vi "SetNeoPixelColourRing.vi"(8 "error in (no error)":errorcluster, 10 "NeoPixel Ring in":T1, 11 "AdaFruit-Seesaw in":refnum<class "AdaFruit-Seesaw.lvclass">) -> (0 "error out":errorcluster, 3 "AdaFruit-Seesaw out":refnum<class "AdaFruit-Seesaw.lvclass">)   [LabVIEW 2020, in "CTI-Scratchpad.lvlib"]
uses:
  CTI-Scratchpad.lvlib
  CTI-Peripheral/AdaFruit-Seesaw/AdaFruit-Seesaw.lvclass
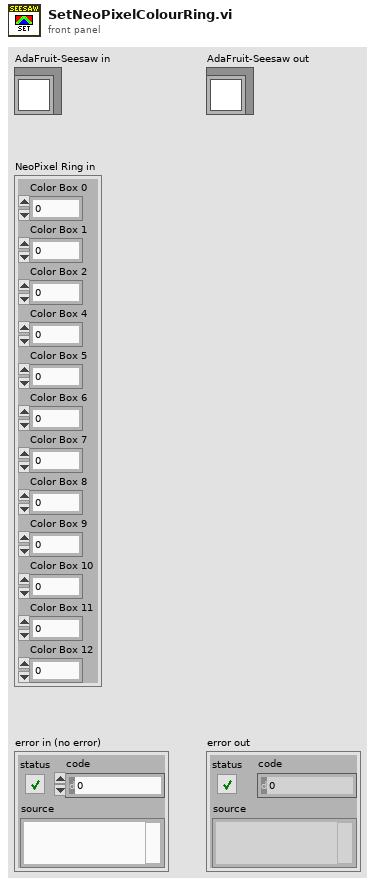
[diagram p1: front panel]
types:
  T1 = cluster{"Color Box 0":u32, "Color Box 1":u32, "Color Box 2":u32, "Color Box 4":u32, "Color Box 5":u32, "Color Box 6":u32, "Color Box 7":u32, "Color Box 8":u32, "Color Box 9":u32, "Color Box 10":u32, "Color Box 11":u32, "Color Box 12":u32}
  T2 = cluster{"Color Box 0":bool, "Color Box 1":bool, "Color Box 2":bool, "Color Box 4":bool, "Color Box 5":bool, "Color Box 6":bool, "Color Box 7":bool, "Color Box 8":bool, "Color Box 9":bool, "Color Box 10":bool, "Color Box 11":bool, "Color Box 12":bool}
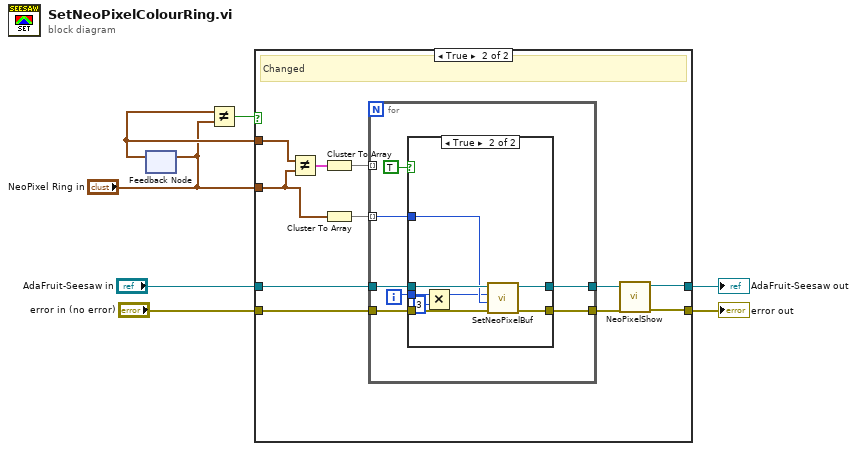
[diagram p0: block diagram]
diagram:
  n1 = feedback-in #1("NeoPixel Ring in") -> ()
  n2 = feedback #1() -> (w2:T1)  [unwired: 1 in]
  n3 = Not Equal?(x=w2, y="NeoPixel Ring in") -> (x != y?=w3:bool)
  n4 = case shown="True" w3 {
    tunnel: [w8 w10] -> w7
    tunnel: [w9 w11] -> w6
    tunnel: "error in (no error)" -> [w8 w20]
    tunnel: "AdaFruit-Seesaw in" -> [w9 w19]
    tunnel: w2 -> [_ w18]
    tunnel: "NeoPixel Ring in" -> [_ w15]
    frame False {
      # "Not Changed - Ignore"
    }
    frame True {
      # "Changed"
      n5 = Not Equal?(x=w18, y=w15) -> (x != y?=w17:T2)
      n6 = Cluster To Array(cluster=w17) -> (array=w16:bool[])
      n7 = Cluster To Array(cluster=w15) -> (array=w14:u32[])
      n8 = for {
        tunnel: w20 -> [w25]
        tunnel: [w27] -> w12
        tunnel: w19 -> [w24]
        tunnel: [w26] -> w13
        tunnel: w16 -> [_] mode=indexing
        tunnel: w14 -> [w23] mode=indexing
        i -> [w22]
        n9 = case shown="True" TRUE {
          tunnel: [w29 w32] -> w27
          tunnel: [w28 w33] -> w26
          tunnel: w25 -> [w29 w37]
          tunnel: w24 -> [w28 w36]
          tunnel: w23 -> [_ w34]
          tunnel: w22 -> [_ w35]
          frame False {
          }
          frame True {
            n10 = Multiply(x=w35, y=3) -> (x*y=w31:i32)
            n11 = call "SetNeoPixelBuf.vi"("error in (no error)"=w37, "Color Box"=w34, "Address"=w31, "AdaFruit-Seesaw in"=w36) -> ("error out"=w32:errorcluster, "AdaFruit-Seesaw out"=w33:refnum<class "AdaFruit-Seesaw.lvclass">)  [unwired: 6 in]
          }
        }
      }
      n12 = call "NeoPixelShow.vi"("error in (no error)"=w12, "AdaFruit-Seesaw in"=w13) -> ("error out"=w10:errorcluster, "AdaFruit-Seesaw out"=w11:refnum<class "AdaFruit-Seesaw.lvclass">)  [unwired: 8 in]
    }
  }
  "error out" <- w7
  "AdaFruit-Seesaw out" <- w6
